vi "CategoryUI.vi"() -> ()   [LabVIEW 2013, in "Category.lvclass"]
doc: "Template for creating new user-interface VIs for inherited classes."
uses:
  Category.lvclass
  <vilib>/NI/AMC/Message Queue.ctl
  <vilib>/NI/AMC/Message.ctl
  <vilib>/NI/Tools/Keyed Array/KeyedArray.ctl
  xCE/xceTreeObj/xceTreeObj.lvclass
  _Shared/Symbols/enum_Symbols.ctl
  Category.lvclass/Category.ctl
  <vilib>/NI/AMC/Read Termination Message.vi
  <vilib>/NI/AMC/Create Single Message.vi
  <vilib>/NI/AMC/Update Message Routing Info.vi
  <vilib>/NI/AMC/Send Message.vi
  <vilib>/NI/AMC/Globals.vi
  <vilib>/NI/AMC/AMC.lvlib
  xCE/xceDataNode/xceDataNode.lvclass
  <vilib>/NI/Tools/Keyed Array/Tools_KeyedArray.lvlib
panel:
  in  "Symbol":T1
  in  "Name":string
  in  "Description":string
  in  "DataNode*":refnum<data-value>
  in  "AMC*":T2
  in  "Exit":bool
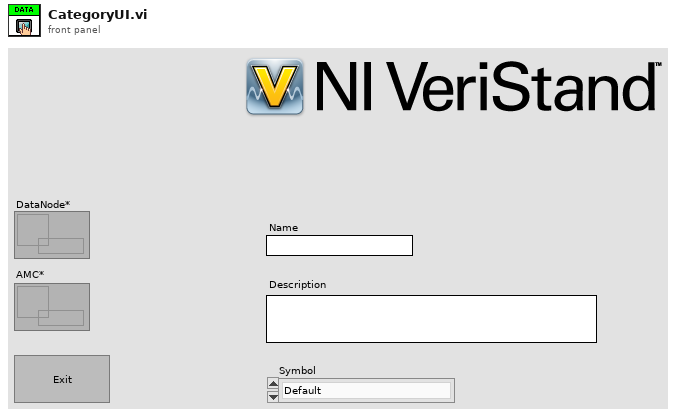
[diagram p1: front panel]
types:
  T1 = typedef "enum_Symbols.ctl" = enum16{"Default", "Analog Input", "Analog Output", "Digital Input", "Digital Output", "PWM Input", "PWM Output"}
  T2 = typedef "AMC.lvlib/Message Queue.ctl" = refnum<queue>
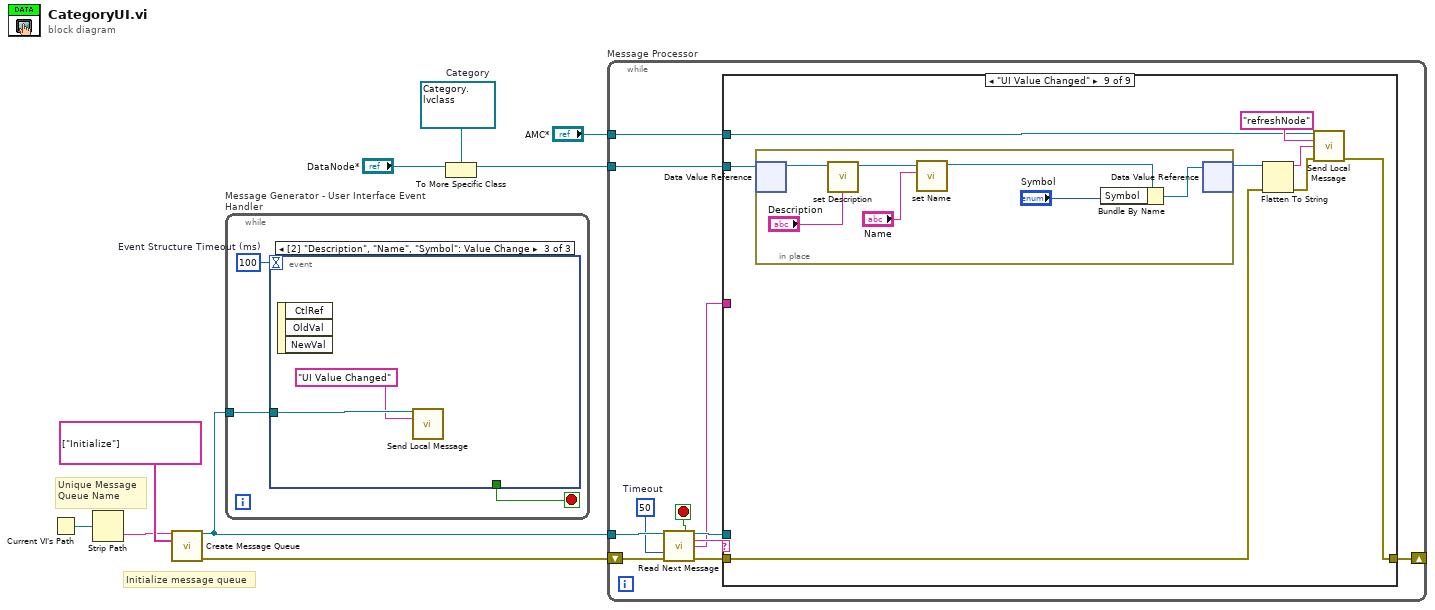
[diagram p0: block diagram]
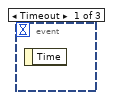
[diagram p2: hidden frame]
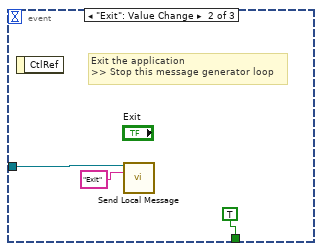
[diagram p3: hidden frame]
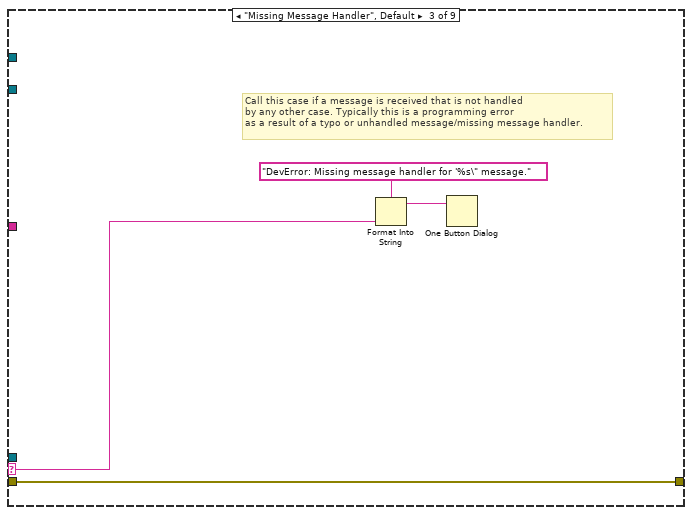
[diagram p6: hidden frame]
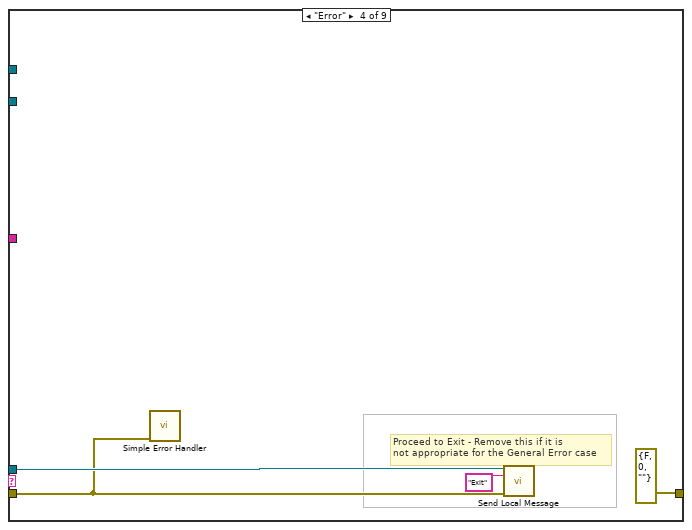
[diagram p7: hidden frame]
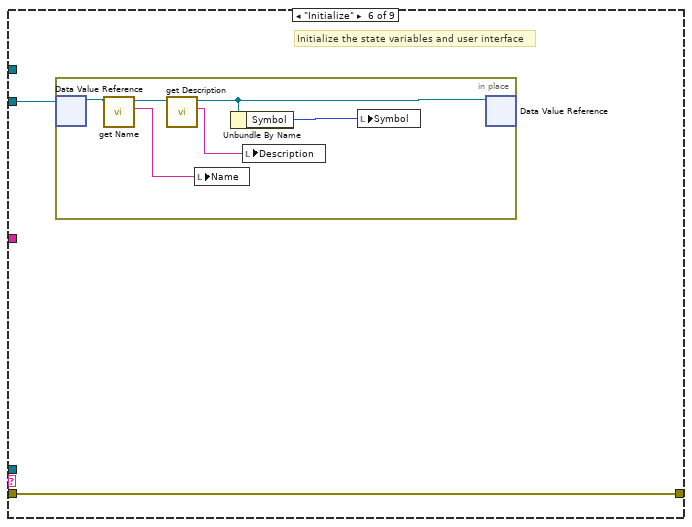
[diagram p9: hidden frame]
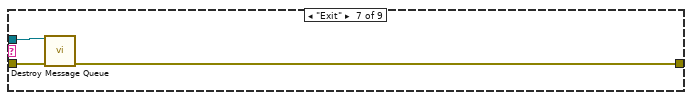
[diagram p10: hidden frame]
diagram:
  w1 = refnum<data-value> refnum  # Category
  # "Initialize message queue"
  # "Unique Message\nQueue Name"
  n1 = Current VI's Path() -> (path=w5:path)
  n2 = Strip Path(path=w5) -> (name=w8:string)  [unwired: 1 out]
  n3 = call <vilib>:"Create Message Queue.vi"("message queue name"=w8, "initial message names"=string[] ["Initialize"]) -> ("message queue out"=w7:T2, "error out"=w6:errorcluster)  [unwired: 12 in]
  n4 = while "Message Generator - User Interface Event Handler" {
    tunnel: w7 -> [w10]
    stop <- w11 stop-if-true
    w12 = 100  # Event Structure Timeout (ms)
    n5 = event shown="[2] \"Description\", \"Name\", \"Symbol\": Value Change" {
      selector: _ -> [_ _ _]
      dyn-events: _ -> [_ _ _]
      timeout: w12 -> [_ _ _]
      tunnel: [_ TRUE ("Discard?") _] -> w11
      tunnel: w10 -> [_ w13 w17]
      event Timeout {
        n6 = event-data() -> ()  [unwired: 2 out]
      }
      event "Exit": Value Change {
        # "Exit the application\n>> Stop this message generator loop"
        n7 = event-data() -> ()  [unwired: 2 out]
        n8 = call <vilib>:"Send Local Message.vi"("message queue in"=w13, "message name"="Exit") -> ()  [unwired: 11 in, 3 out]
      }
      event "Description", "Name": Value Change {
        n9 = event-data() -> ()  [unwired: 4 out]
        n10 = call <vilib>:"Send Local Message.vi"("message queue in"=w17, "message name"="UI Value Changed" ("Message Name")) -> ()  [unwired: 11 in, 3 out]
      }
    }
  }
  n11 = To More Specific Class(target class=w1, reference="DataNode*") -> (specific class reference=w2:refnum<data-value>)  [unwired: 1 in, 1 out]
  n12 = while "Message Processor" {
    shift-left: w6 -> [w24]
    shift-right: [w28] -> _
    tunnel: w7 -> [w25]
    tunnel: "AMC*" -> [w18]
    tunnel: w2 -> [w19]
    stop <- w27 stop-if-true
    w22 = 50  # Timeout
    n13 = call <vilib>:"Read Next Message.vi"("message queue in"=w25, "timeout (1 ms)"=w22, "error in"=w24) -> ("exit process?"=w27:bool, "message queue out"=w26:T2, "message name"=w21:string, "message value"=w20:string, "error out"=w23:errorcluster)  [unwired: 5 in, 3 out]
    n14 = case shown="\"UI Value Changed\"" w21 {
      selector: w21 -> [_ _ w33 _ _ _ _ _ _]
      tunnel: w26 -> [_ _ _ w37 _ _ w49 _ _]
      tunnel: w23 -> [w29 w30 w34 w35 w39 w41 w50 w51 w53]
      tunnel: [w29 w30 w34 errorcluster {"status"=FALSE, "code"=0, "source"=""} ("error out") w39 w41 w48 w51 w52] -> w28
      tunnel: w20 -> [_ _ _ _ _ _ _ _ _]
      tunnel: w19 -> [_ _ _ _ _ w40 _ _ w59]
      tunnel: w18 -> [_ _ _ _ _ _ _ _ w55]
      frame "---------- Framework Operations ----------" {
        # "Dummy case to add a seperator in the Case Structure menu"
      }
      frame "", "Idle" {
      }
      frame "Missing Message Handler", Default {
        # "Call this case if a message is received that is not handled \nby any other case. Typically this is a programming error\nas a result of a typo or unhandled message/missing message handler."
        n15 = Format Into String(format string="DevError: Missing message handler for '%s\" message." ("message"), w33) -> (resulting string=w31:string)  [unwired: 2 in, 1 out]
        n16 = One Button Dialog(message=w31) -> ()  [unwired: 2 out]
      }
      frame "Error" {
        # "Proceed to Exit - Remove this if it is\nnot appropriate for the General Error case"
        n17 = call <vilib>:"Simple Error Handler.vi"("error in (no error)"=w35) -> ()  [unwired: 1 in, 8 out]
        n18 = call <vilib>:"Send Local Message.vi"("message queue in"=w37, "message name"="Exit", "error in"=w35) -> ()  [unwired: 10 in, 3 out]
      }
      frame "---------- Generic Operations ----------" {
        # "Dummy case to add a seperator in the Case Structure menu"
      }
      frame "Initialize" {
        # "Initialize the state variables and user interface"
        n19 = in-place {
          n20 = in-place-dvr #1(w40) -> (w47:refnum<class "Category.lvclass">)  [unwired: 1 out]
          n21 = call "get Name.vi"("xceDataNode in"=w47) -> ("Name"=w44:string, "xceDataNode out"=w46:refnum<class "Category.lvclass">)  [unwired: 8 in, 1 out]
          n22 = call "get Description.vi"("xceDataNode in"=w46) -> ("Description"=w45:string, "xceDataNode out"=w43:refnum<class "Category.lvclass">)  [unwired: 8 in, 1 out]
          n23 = local write "Name"(w44) -> ()
          n24 = Unbundle By Name(w43) -> ("Symbol"=w42:T1)
          n25 = local write "Description"(w45) -> ()
          n26 = local write "Symbol"(w42) -> ()
          n27 = in-place-dvr #1(w43) -> ()  [unwired: 2 out]
        }
      }
      frame "Exit" {
        n28 = call <vilib>:"Destroy Message Queue.vi"("message queue in"=w49, "error in"=w50) -> ("error out"=w48:errorcluster)  [unwired: 11 in, 2 out]
      }
      frame "---------- Application Operations ----------" {
        # "Dummy case to add a seperator in the Case Structure menu"
      }
      frame "UI Value Changed" {
        n29 = in-place {
          n30 = in-place-dvr #2(w59) -> (w65:refnum<class "Category.lvclass">)  [unwired: 1 out]
          n31 = call "set Description.vi"("Description"="Description", "xceDataNode in"=w65) -> ("xceDataNode out"=w63:refnum<class "Category.lvclass">)  [unwired: 8 in, 1 out]
          n32 = call "set Name.vi"("Name"="Name", "xceDataNode in"=w63) -> ("xceDataNode out"=w62:refnum<class "Category.lvclass">)  [unwired: 8 in, 1 out]
          n33 = Bundle By Name(cluster=w62, "Symbol"="Symbol") -> (w66:refnum<class "Category.lvclass">)
          n34 = in-place-dvr #2(w66) -> (w54:refnum<data-value>)  [unwired: 1 out]
        }
        n35 = Flatten To String(anything=w54, error in (no error)=w53) -> (data string=w58:string, error out=w56:errorcluster)  [unwired: 2 in, 1 out]
        n36 = call <vilib>:"Send Local Message.vi"("message queue in"=w55, "message name"="refreshNode" ("Message Name"), "message value"=w58, "error in"=w56) -> ("error out"=w52:errorcluster)  [unwired: 9 in, 2 out]
      }
    }
  }
